vi "IgnitionTest.vi"() -> ()   [LabVIEW 2017]
panel:
  in  "PT Filename":path=path "ignitiontest-pt.xlsx" caption="Filename"
  in  "Stop PT":bool
  out "Pressure (psi)":dynamicdata(graph)
  out "Thermocouples":dbl[](array[numeric])
  in  "Stop TC":bool
  in  "TC Filename":path=path "ignitiontest-tc.xlsx" caption="Filename"
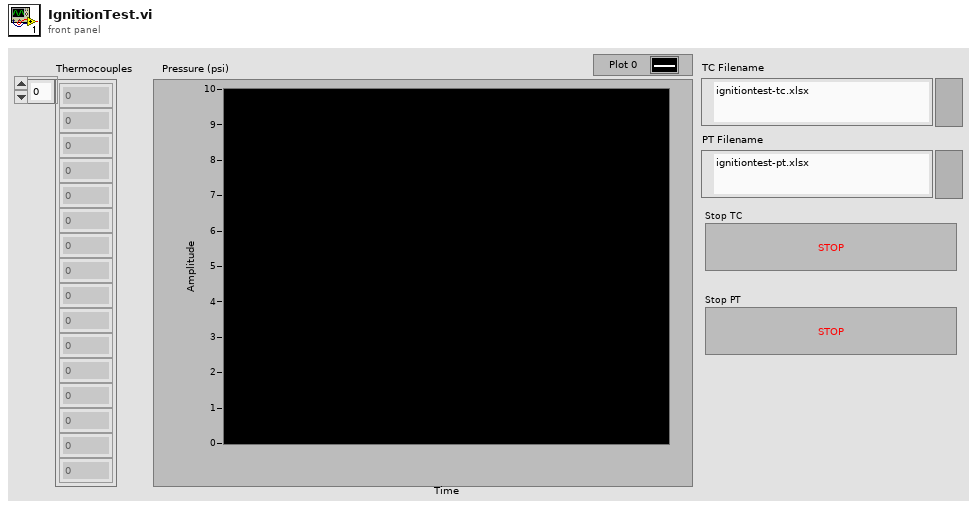
[diagram p1: front panel]
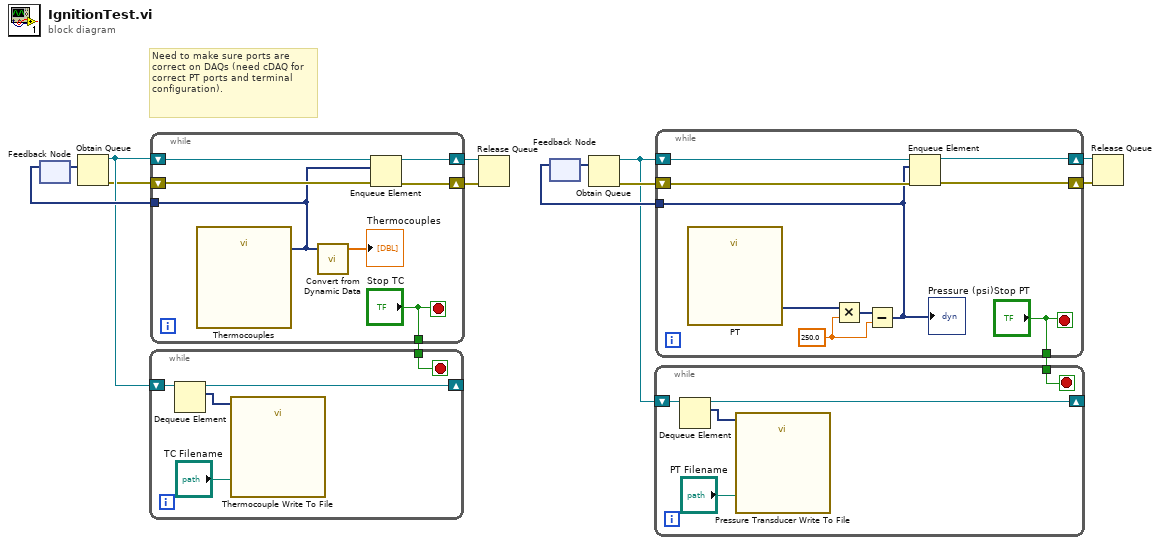
[diagram p0: block diagram]
diagram:
  # "Need to make sure ports are correct on DAQs (need cDAQ for correct PT ports and terminal configuration)."
  n1 = feedback #1() -> (w13:dynamicdata)  [unwired: 1 in]
  n2 = Obtain Queue(element data type=w13) -> (queue out=w10:refnum<queue>, error out=w9:errorcluster)  [unwired: 4 in, 1 out]
  n3 = while {
    tunnel: [w18] -> w14
    shift-right: [w17] -> w12
    shift-left: w10 -> [w19]
    shift-right: [w16] -> w11
    shift-left: w9 -> [w20]
    tunnel: ["Stop TC"] -> w8
    stop <- "Stop TC" stop-if-true
    n4 = call "Thermocouples"() -> ("data"=w18:dynamicdata)  [unwired: 16 in, 3 out]
    n5 = call "Convert from Dynamic Data"("Dynamic Data Type"=w18) -> ("Array"=→"Thermocouples":dbl[])  [unwired: 3 in]
    n6 = Enqueue Element(queue=w19, element=w18, error in (no error)=w20) -> (queue out=w17:refnum<queue>, error out=w16:errorcluster)  [unwired: 1 in, 1 out]
  }
  n7 = feedback-in #1(w14) -> ()
  n8 = while {
    shift-right: [w24] -> _
    shift-left: w10 -> [w25]
    tunnel: w8 -> [w23]
    stop <- w23 stop-if-true
    n9 = Dequeue Element(queue=w25) -> (queue out=w24:refnum<queue>, element=w22:dynamicdata)  [unwired: 2 in, 2 out]
    n10 = call "Thermocouple Write To File"("Signals"=w22, "Filename"="TC Filename") -> ()  [unwired: 15 in, 3 out]
  }
  n11 = Release Queue(queue=w12, error in (no error)=w11) -> ()  [unwired: 1 in, 3 out]
  n12 = feedback #2() -> (w3:dynamicdata)  [unwired: 1 in]
  n13 = Obtain Queue(element data type=w3) -> (queue out=w2:refnum<queue>, error out=w5:errorcluster)  [unwired: 4 in, 1 out]
  n14 = while {
    shift-right: [w31] -> w7
    shift-left: w2 -> [w32]
    shift-right: [w29] -> w6
    shift-left: w5 -> [w30]
    tunnel: [w28] -> w4
    tunnel: ["Stop PT"] -> w1
    stop <- "Stop PT" stop-if-true
    w34 = 250.0
    n15 = call "PT"() -> ("data"=w33:dynamicdata)  [unwired: 16 in, 3 out]
    n16 = Multiply(x=w33, y=w34) -> (x*y=w35:dynamicdata)
    n17 = Subtract(x=w35, y=w34) -> (x-y=w28:dynamicdata)
    "Pressure (psi)" <- w28
    n18 = Enqueue Element(queue=w32, element=w28, error in (no error)=w30) -> (queue out=w31:refnum<queue>, error out=w29:errorcluster)  [unwired: 1 in, 1 out]
  }
  n19 = feedback-in #2(w4) -> ()
  n20 = while {
    shift-right: [w38] -> _
    shift-left: w2 -> [w39]
    tunnel: w1 -> [w37]
    stop <- w37 stop-if-true
    n21 = Dequeue Element(queue=w39) -> (queue out=w38:refnum<queue>, element=w36:dynamicdata)  [unwired: 2 in, 2 out]
    n22 = call "Pressure Transducer Write To File"("Signals"=w36, "Filename"="PT Filename") -> ()  [unwired: 15 in, 3 out]
  }
  n23 = Release Queue(queue=w7, error in (no error)=w6) -> ()  [unwired: 1 in, 3 out]
